vi "DefBallOrientSkill.vi"(8 "error in (no error)":errorcluster, 9 "Robot":refnum<class "Robot.lvclass">, 10 "Game":refnum<class "Game.lvclass">, 11 "DefBallOrientSkill in":refnum<class "DefBallOrientSkill.lvclass">) -> (0 "error out":errorcluster, 2 "Robot out":refnum<class "Robot.lvclass">, 3 "DefBallOrientSkill out":refnum<class "DefBallOrientSkill.lvclass">)   [LabVIEW 2023, in "DefBallOrientSkill.lvclass"]
uses:
  DefBallOrientSkill.lvclass
  Game_class/Game.lvclass
  Robot_class/Robot.lvclass
  Game_class/Game.lvclass/Game.ctl
  Referee_class/Referee.lvclass/Referee.ctl
  Parameters_class/Parameters.lvclass/Parameters.ctl
  Team_class/Team.lvclass/Team.ctl
  Object_class/Object.lvclass/Object.ctl
  Robot_class/Robot.lvclass/Robot.ctl
  Game_class/Read BallRef.vi
  Object_class/Read x.vi
  Object_class/Read y.vi
  Game_class/Read Referee.vi
  Game_class/Read Parameters.lvclass.vi
  Game_class/Read FieldRef.vi
  Game_class/Read Utilities.lvclass.vi
  Game_class/Read AllyRef.vi
  Game_class/Read EnemyRef.vi
  Team_class/Read RobotRef.vi
  Parameters_class/Read GoalieInFrontGoal.vi
  Parameters_class/Read AttakingOurselves.vi
  Referee_class/Read our_goalie_id.vi
  Robot_class/Read orientation.vi
  Robot_class/Write dest_x.vi
  Robot_class/Write dest_y.vi
  Robot_class/Write dest_orientation.vi
  Enemy_class/Enemy.lvclass
  Ally_class/Ally.lvclass
  Ball_class/Ball.lvclass
  Referee_class/Referee.lvclass
  Parameters_class/Parameters.lvclass
  Field_class/Field.lvclass
  Utilities_class/Utilities.lvclass
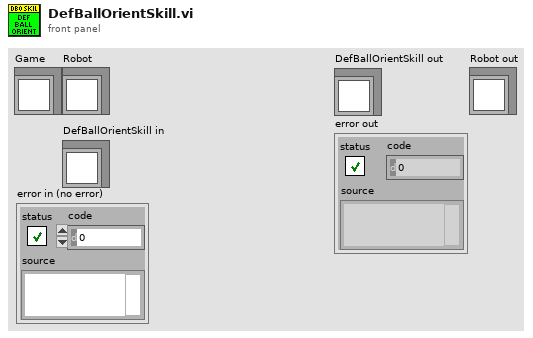
[diagram p1: front panel]
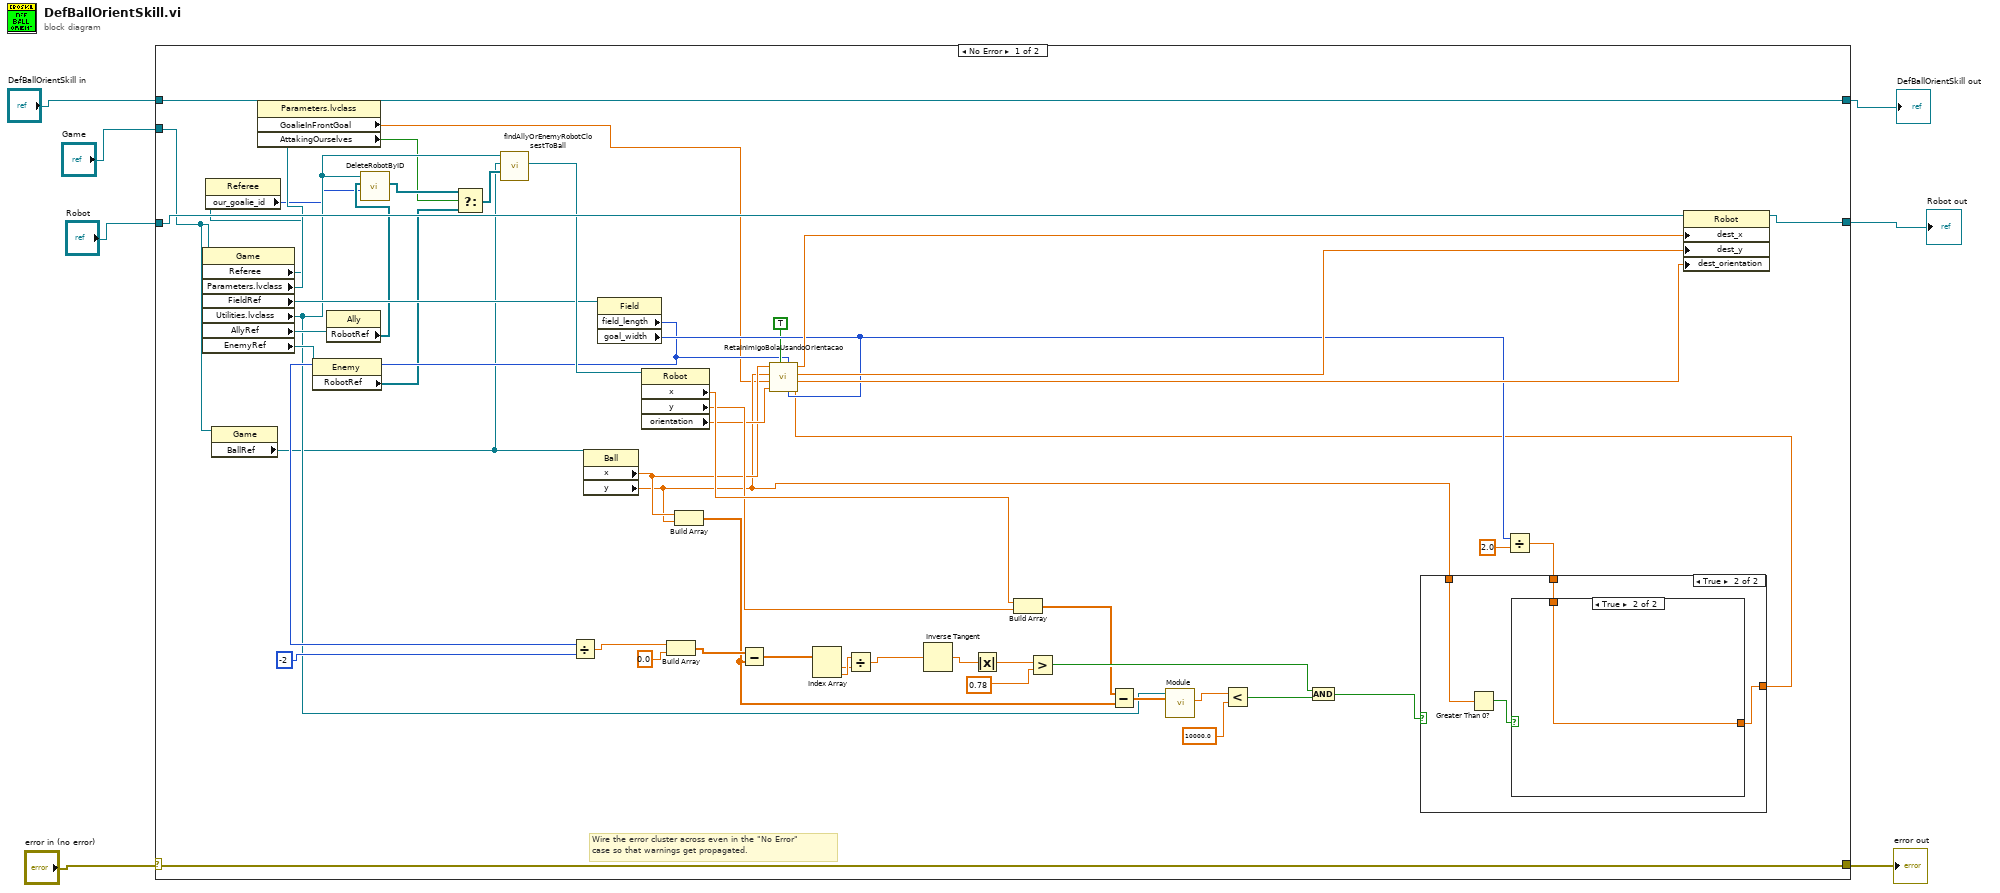
[diagram p0: block diagram]
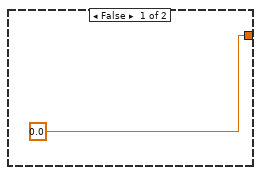
[diagram p2: hidden frame]
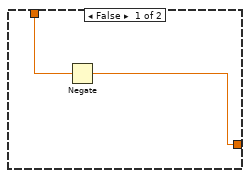
[diagram p3: hidden frame]
diagram:
  n1 = case shown="No Error" "error in (no error)" {
    selector: "error in (no error)" -> [w59 w70]
    tunnel: [w59 w70] -> w2
    tunnel: [w60 w69] -> w6
    tunnel: "DefBallOrientSkill in" -> [w60 w69]
    tunnel: "Robot" -> [w58 _]
    tunnel: "Game" -> [w21 _]
    tunnel: [w32 _] -> w1
    frame No Error {
      # "Wire the error cluster across even in the \"No Error\"\ncase so that warnings get propagated."
      n2 = property class="Game"(reference=w21) -> ("Referee"=w12:refnum<class "Referee.lvclass">, "Parameters.lvclass"=w20:refnum<class "Parameters.lvclass">, "FieldRef"=w56:refnum<class "Field.lvclass">, "Utilities.lvclass"=w14:refnum<class "Utilities.lvclass">, "AllyRef"=w19:refnum<class "Ally.lvclass">, "EnemyRef"=w18:refnum<class "Enemy.lvclass">)  [unwired: 1 in, 2 out]
      n3 = property class="Referee"(reference=w12) -> ("our_goalie_id"=w11:i32)  [unwired: 1 in, 2 out]
      n4 = property class="Game"(reference=w21) -> ("BallRef"=w8:refnum<class "Ball.lvclass">)  [unwired: 1 in, 2 out]
      n5 = property class="Parameters.lvclass"(reference=w20) -> ("GoalieInFrontGoal"=w9:dbl, "AttakingOurselves"=w10:bool)  [unwired: 1 in, 2 out]
      n6 = property class="Enemy"(reference=w18) -> ("RobotRef"=w17:refnum<class "Robot.lvclass">[])  [unwired: 1 in, 2 out]
      n7 = property class="Ally"(reference=w19) -> ("RobotRef"=w13:refnum<class "Robot.lvclass">[])  [unwired: 1 in, 2 out]
      n8 = call-dynamic "DeleteRobotByID.vi"("id"=w11, "RobotRef"=w13, "Utilities in"=w14) -> ("RobotRef out"=w15:refnum<class "Robot.lvclass">[])  [unwired: 6 in, 2 out]
      n9 = Select(t=w15, s=w10, f=w17) -> (s? t:f=w16:refnum<class "Robot.lvclass">[])
      n10 = call "findAllyOrEnemyRobotClosestToBall.vi"("Ally/Enemy Robots"=w16, "Ball"=w8, "Utilities in"=w14) -> ("Robot"=w57:refnum<class "Robot.lvclass">)  [unwired: 5 in, 3 out]
      n11 = property class="Ball"(reference=w8) -> ("x"=w25:dbl, "y"=w24:dbl)  [unwired: 1 in, 2 out]
      n12 = property class="Field"(reference=w56) -> ("field_length"=w22:i32, "goal_width"=w28:i32)  [unwired: 1 in, 2 out]
      n13 = Divide(x=w22, y=-2) -> (x/y=w48:dbl)
      n14 = property class="Robot"(reference=w57) -> ("x"=w36:dbl, "y"=w35:dbl, "orientation"=w26:dbl)  [unwired: 1 in, 2 out]
      n15 = Build Array(w48, 0.0 ("element")) -> (w51:dbl[])
      n16 = Build Array(w25, w24) -> (w33:dbl[])
      n17 = Subtract(x=w51, y=w33) -> (x-y=w50:dbl[])
      n18 = Index Array(array=w50) -> (element #1=w46:dbl, element #2=w47:dbl)  [unwired: 2 in]
      n19 = Divide(x=w47, y=w46) -> (x/y=w45:dbl)
      n20 = Inverse Tangent(1:w45) -> (0:w44:dbl)
      n21 = Absolute Value(x=w44) -> (abs(x)=w49:dbl)
      n22 = Build Array(w36, w35) -> (w34:dbl[])
      n23 = Greater?(x=w49, y=0.78) -> (0:w40:bool)
      n24 = Subtract(x=w34, y=w33) -> (x-y=w38:dbl[])
      n25 = call-dynamic "Module.vi"("2D vector"=w38, "Utilities in"=w14) -> ("Modulo"=w37:dbl)  [unwired: 7 in, 2 out]
      n26 = Less?(x=w37, y=10000.0) -> (x < y?=w41:bool)
      n27 = And(x=w40, y=w41) -> (x .and. y?=w39:bool)
      n28 = Divide(x=w28, y=2.0) -> (x/y=w55:dbl)
      n29 = case shown="True" w39 {
        tunnel: w55 -> [_ w64]
        tunnel: [0.0 w63] -> w27
        tunnel: w24 -> [_ w62]
        frame False {
        }
        frame True {
          n30 = Greater Than 0?(x=w62) -> (x > 0?=w65:bool)
          n31 = case shown="True" w65 {
            tunnel: w64 -> [w67 w68]
            tunnel: [w66 w68] -> w63
            frame False {
              n32 = Negate(x=w67) -> (-x=w66:dbl)
            }
            frame True {
            }
          }
        }
      }
      n33 = call "RetaInimigoBolaUsandoOrientacao.vi"("Y quina"=w27, "Goal Width"=w28, "Field length"=w22, "Meio?"=TRUE, "Orientação inimigo"=w26, "DistDistInFrontGoal"=w9, "Y bola"=w24, "X bola"=w25) -> ("Orientação goleiro"=w29:dbl, "Y golerio"=w30:dbl, "X goleiro"=w31:dbl)  [unwired: 1 in]
      n34 = property class="Robot"(reference=w58, "dest_x"=w31, "dest_y"=w30, "dest_orientation"=w29) -> (reference out=w32:refnum<class "Robot.lvclass">)  [unwired: 1 in, 1 out]
    }
    frame Error {
    }
  }
  "DefBallOrientSkill out" <- w6
  "error out" <- w2
  "Robot out" <- w1
